vi "Unpack Control Mouse Up.vi"(11 "ControlMouseUpMsg":refnum<class "ControlMouseUpMsg.lvclass">) -> (0 "Button":u16, 1 "Coords":T2, 2 "Time":u32, 3 "Control Label":string, 4 "Mods":cluster{"Double Click":bool, "Menu Key":bool}, 5 "Ctl Refnum":refnum<vi>, 6 "PlatMods":T1)   [LabVIEW 2017, in "ActorEvents.lvlib" / "ControlMouseUpMsg.lvclass"]
doc: "<License>\nCopyright © 2017 Composed Systems, LLC | All rights reserved\nwww.composed.io\n\nAuthor: Ethan Stern <ethan.stern@composed.io>\n\nThis software is provided \"AS IS\" WITHOUT WARRANTIES, either express or implied, AND IS FOR EDUCATIONAL PURPOSES ONLY.\n</License>"
uses:
  <vilib>/gpm_packages/@cs/mva-viewable/Source/ActorEvents/IEventAggregator Messages/ControlMouseUpMsg/ControlMouseUpMsg.lvclass
  <vilib>/Utility/miscctls.llb/LVPoint32TypeDef.ctl
  <vilib>/gpm_packages/@cs/mva-viewable/Source/ActorEvents/IEventAggregator Messages/ControlMouseUpMsg/ControlMouseUpMsg.lvclass/ControlMouseUpMsg.ctl
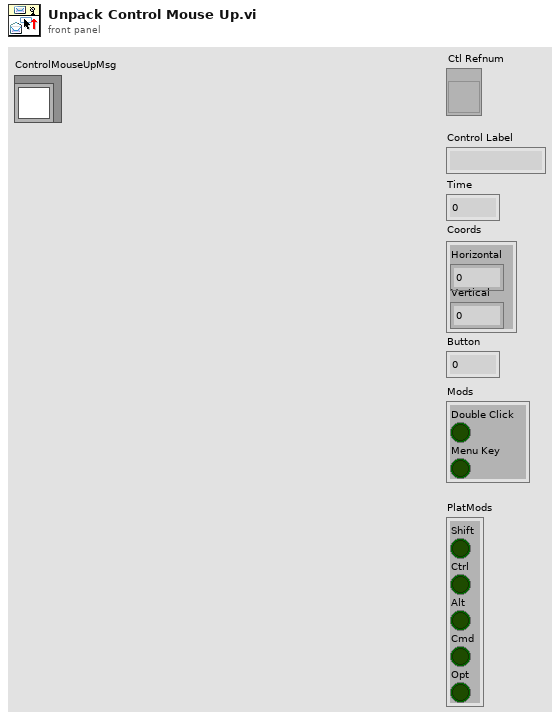
[diagram p1: front panel]
types:
  T1 = cluster{"Shift":bool, "Ctrl":bool, "Alt":bool, "Cmd":bool, "Opt":bool}
  T2 = typedef "LVPoint32TypeDef.ctl" = cluster{"Horizontal":i32, "Vertical":i32}
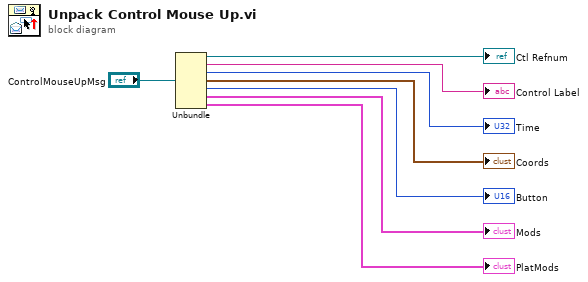
[diagram p0: block diagram]
diagram:
  n1 = Unbundle("ControlMouseUpMsg") -> (→"Ctl Refnum":refnum<vi>, →"Control Label":string, →"Time":u32, →"Coords":T2, →"Button":u16, →"Mods":cluster{"Double Click":bool, "Menu Key":bool}, →"PlatMods":T1)
